vi "PathPlanner_PathFinder_ClearRHS.vi"() -> (3 "Rhs":map{i32, dbl}(c390))   [LabVIEW 2019]
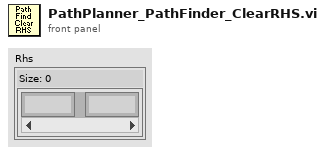
[diagram p1: front panel]
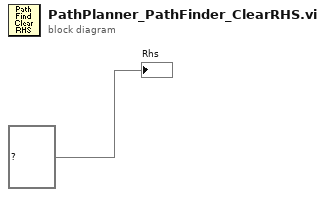
[diagram p0: block diagram]
diagram:
  "Rhs" <- map{i32, dbl} {} ("Rhs")
